vi "Record QPD-three axis.vi"() -> ()   [LabVIEW 2014]
uses:
  <vilib>/Analysis/baseanly.llb/Mean (DBL).vi
  <vilib>/Analysis/NI_AALBase.lvlib
panel:
  out "QPD-z":dbl(graph)
  out "QPD-y":dbl(graph)
  out "QPD-x":dbl(graph)
  in  "number of samples":i32=500
  in  "rate":dbl=30000.0
  in  "stop":bool
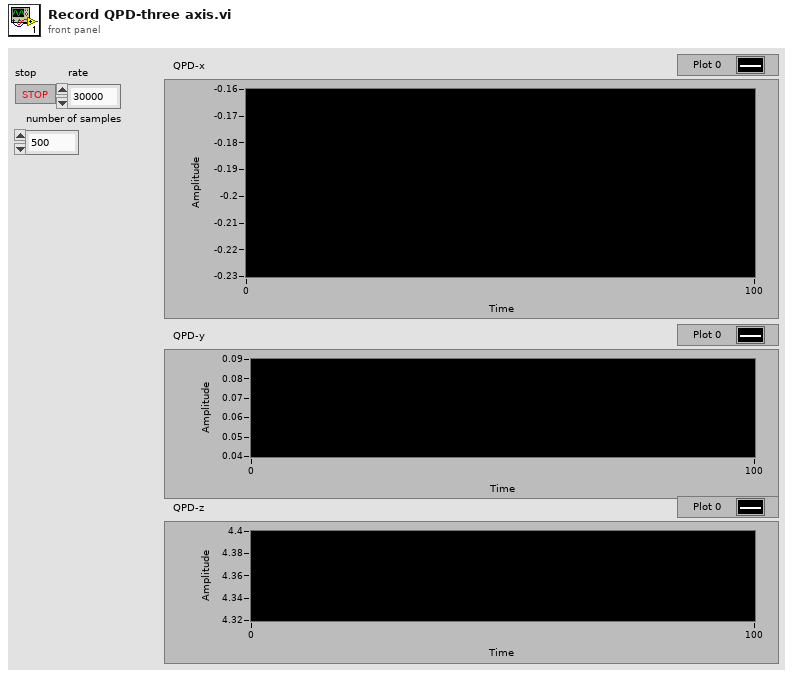
[diagram p1: front panel]
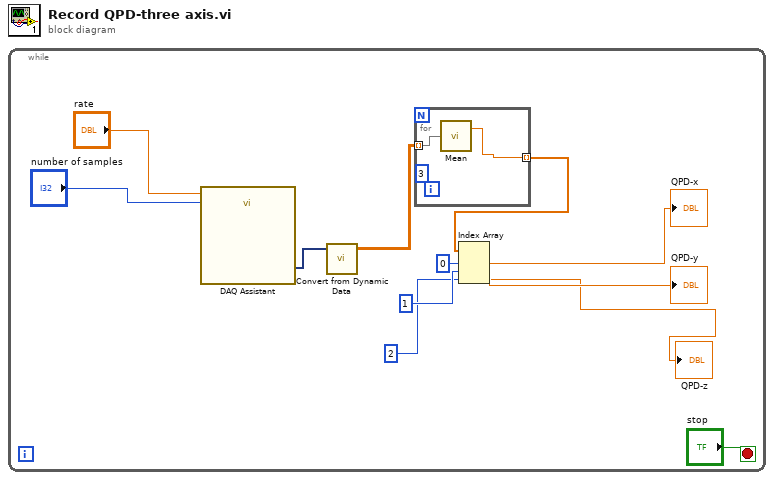
[diagram p0: block diagram]
diagram:
  n1 = while {
    stop <- "stop" stop-if-true
    n2 = call "DAQ Assistant"("rate"="rate", "number of samples"="number of samples") -> ("data"=w9:dynamicdata)  [unwired: 14 in, 3 out]
    n3 = call "Convert from Dynamic Data"("Dynamic Data Type"=w9) -> ("Array"=w5:dbl[][])  [unwired: 3 in]
    n4 = for {
      tunnel: w5 -> [w14] mode=indexing
      tunnel: [w13] -> w4 mode=indexing
      (unwired) 3 ("polynomial order")
      n5 = call-poly <vilib>:"Mean.vi"("X"=w14) -> ("mean"=w13:dbl)  [unwired: 1 out]
    }
    n6 = Index Array(array=w4, index #1=0 ("index (row)"), index #2=1 ("index (row)"), index #3=2 ("index (row)")) -> (element #1=→"QPD-x":dbl, element #2=→"QPD-y":dbl, element #3=→"QPD-z":dbl)
  }
